vi "Write Sample.vi"(8 "error in (no error)":errorcluster, 10 "Sample":refnum<class "Sample.lvclass">, 11 "Syringe Line in":refnum<class "Syringe Line.lvclass">) -> (0 "error out":errorcluster, 3 "Syringe Line out":refnum<class "Syringe Line.lvclass">)   [LabVIEW 2015, in "cRIO-Carbondioxide.lvlib" / "CO2-Actor.lvlib" / "Syringe Line.lvclass"]
uses:
  Syringe Line.lvclass
  subs/Sample/Sample.lvclass
  Syringe Line.lvclass/Syringe Line.ctl
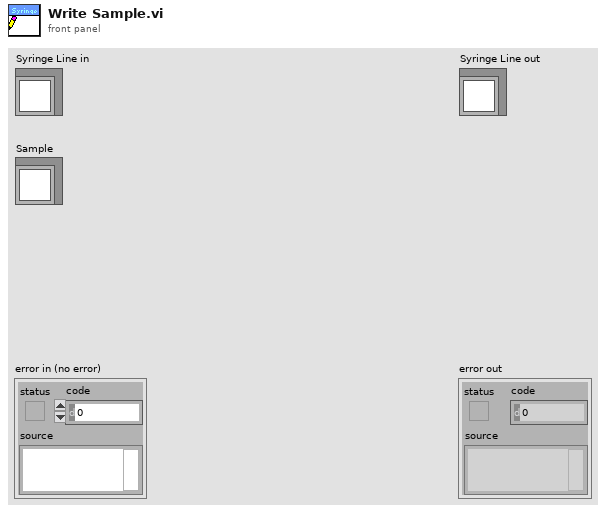
[diagram p1: front panel]
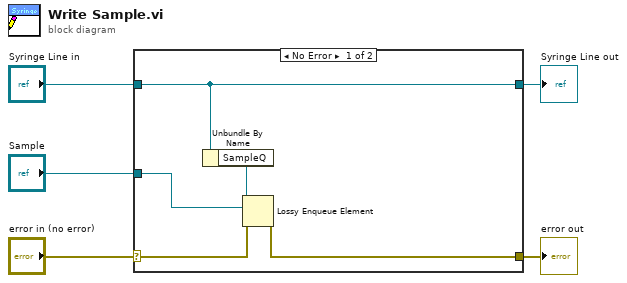
[diagram p0: block diagram]
diagram:
  n1 = case shown="No Error" "error in (no error)" {
    selector: "error in (no error)" -> [w8 w11]
    tunnel: [w7 w11] -> w4
    tunnel: [w6 w12] -> w2
    tunnel: "Syringe Line in" -> [w6 w12]
    tunnel: "Sample" -> [w10 _]
    frame No Error {
      n2 = Unbundle By Name(w6) -> ("SampleQ"=w9:refnum<queue>)
      n3 = Lossy Enqueue Element(queue=w9, element=w10, error in (no error)=w8) -> (error out=w7:errorcluster)  [unwired: 3 out]
    }
    frame Error {
    }
  }
  "error out" <- w4
  "Syringe Line out" <- w2
